vi "snaps of BD AND FP.vi"() -> ()   [LabVIEW 2018]
panel:
  in  "Boolean":bool
  out "Tank":dbl(slide) scale=0.0..10.0
  out "Gauge":dbl(knob) scale=0.0..100.0
  in  "Knob":dbl(knob) scale=0.0..100.0
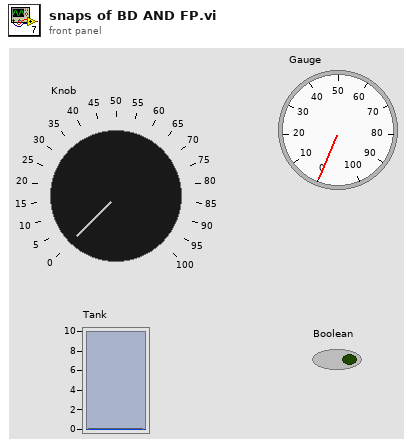
[diagram p1: front panel]
types:
  T1 = typedef "imagedata.ctl" = cluster{"image type":i32, "image depth":i32, "image":u8[], "mask":u8[], "colors":u32[], "Rectangle":cluster{"left":i16, "top":i16, "right":i16, "bottom":i16}}
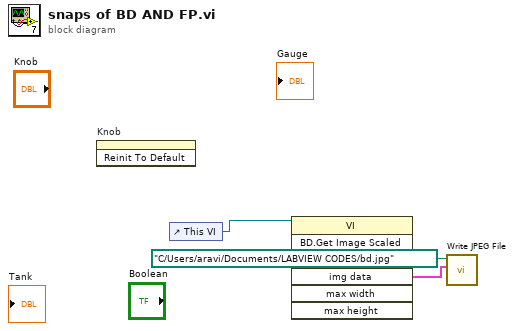
[diagram p0: block diagram]
diagram:
  n1 = invoke on="Knob" class="Knob (strict)" method="Reinit To Default"() -> ()  [unwired: 3 in, 3 out]
  n2 = control-ref of="This VI"() -> (w3:refnum<vi>)
  n3 = invoke class="VI" method="BD.Get Image Scaled"(reference=w3) -> ("img data"=w1:T1)  [unwired: 6 in, 6 out]
  n4 = call <vilib>:"Write JPEG File.vi"("image data"=w1, "path to JPEG file"=path "C:/Users/aravi/Documents/LABVIEW CODES/bd.jpg") -> ()  [unwired: 8 in, 2 out]
